vi "SubVI_ProcessImage.vi"(0 "Image Path":path, 1 "Path to Python.exe":path=path "Python", 2 "Initial Guess":T1={"Center (pixels)"=-1.0, "Reflectivity"=0.0} {"Center (pixels)" format="%#_16g"}) -> (3 "Success":bool, 4 "Params Vector":dbl[](array[numeric]) format="%#_10f", 5 "Errors":dbl[](array[numeric]) format="%#_2g", 6 "Iterations":i32)   [LabVIEW 2016]
panel:
  out "error out":errorcluster
  out "Graph of Final Fit":cluster{dbl[], dbl[]}[](graph) caption="XY Graph"
  out "standard error":string
  out "return code":i32
  # "1. Imputs"
  # "2. Outputs"
  # "Center (px)"
  # "Reflectivity (ul)"
  # "Amplitude (px val^2)"
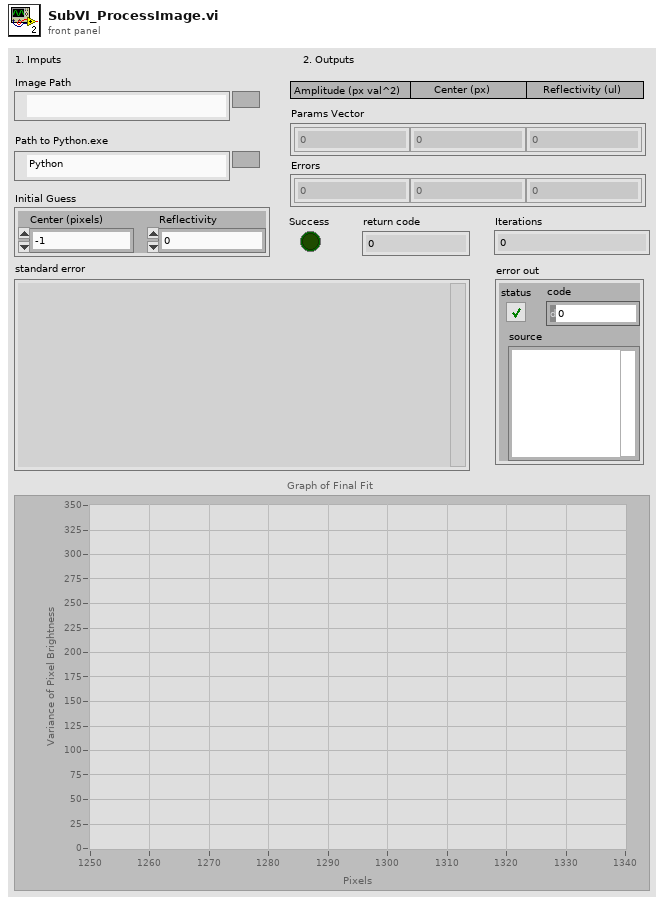
[diagram p1: front panel]
types:
  T1 = cluster{"Center (pixels)":dbl, "Reflectivity":dbl}
  T2 = cluster{"Image Path":path, "Initial Guess":cluster{"Center (pixels)":dbl, "Reflectivity":dbl}}
  T3 = cluster{dbl[], dbl[], i32, cluster{dbl[], dbl[], dbl[]}}
  T4 = enum8{"Enabled", "Disabled", "Disabled and Grayed Out"}
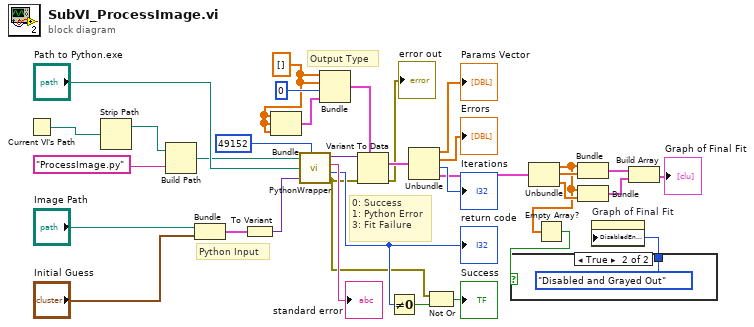
[diagram p0: block diagram]
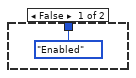
[diagram p2: hidden frame]
diagram:
  w14 = dbl[] []
  # "0: Success\n1: Python Error\n3: Fit Failure"
  # "Python Input"
  # "Output Type"
  n1 = Current VI's Path() -> (path=w34:path)
  n2 = Strip Path(path=w34) -> (stripped path=w21:path)  [unwired: 1 out]
  n3 = Build Path(base path=w21, name or relative path="ProcessImage.py") -> (appended path=w22:path)
  n4 = Bundle("Image Path"="Image Path", "Initial Guess"="Initial Guess") -> (w20:T2)  [unwired: 1 in]
  n5 = To Variant(anything=w20) -> (Variant=w31:variant)
  n6 = Bundle(w14, w14, w14) -> (w15:cluster{dbl[], dbl[], dbl[]})  [unwired: 1 in]
  n7 = call "PythonWrapper.vi"("file to run"=w22, "expected output size (4096)"=u32 49152, "Python.exe"="Path to Python.exe", "data in"=w31) -> ("data out"=w29:variant, "standard error"=→"standard error":string, "return code"=w18:i32, "error out"=w1:errorcluster)  [unwired: 1 in]
  "return code" <- w18
  n8 = Bundle(w14, w14, 0, w15) -> (w27:T3)  [unwired: 1 in]
  n9 = Variant To Data(error in=w1, type=w27, Variant=w29) -> (data=w26:T3, error out=→"error out":errorcluster)
  n10 = Not Equal To 0?(x=w18) -> (x != 0?=w2:bool)
  n11 = Unbundle(w26) -> (→"Params Vector":dbl[], →"Errors":dbl[], →"Iterations":i32, w13:cluster{dbl[], dbl[], dbl[]})
  n12 = Not Or(1:w2, 2:w1) -> (0:→"Success":bool)
  n13 = Unbundle(w13) -> (w6:dbl[], w12:dbl[], w11:dbl[])
  n14 = Empty Array?(array=w6) -> (empty?=w5:bool)
  n15 = case shown="True" w5 {
    tunnel: [T4."Enabled" ("Disabled") T4."Disabled and Grayed Out" ("Disabled")] -> w7
    frame False {
    }
    frame True {
    }
  }
  n16 = Bundle(w6, w12) -> (w9:cluster{dbl[], dbl[]})  [unwired: 1 in]
  n17 = Bundle(w6, w11) -> (w8:cluster{dbl[], dbl[]})  [unwired: 1 in]
  n18 = property on="Graph of Final Fit" class="XYGraph (strict)"("DisabledEnum"=w7) -> ()  [unwired: 2 in, 2 out]
  n19 = Build Array(w9, w8) -> (→"Graph of Final Fit":cluster{dbl[], dbl[]}[])
